vi "例程02-并行转顺序、基于数据流运行.vi"() -> ()   [LabVIEW 2018]
panel:
  out "结果显示 2":dbl
  in  "输入4":dbl
  in  "输入3":dbl
  out "结果显示":dbl
  in  "输入2":dbl
  in  "输入1":dbl
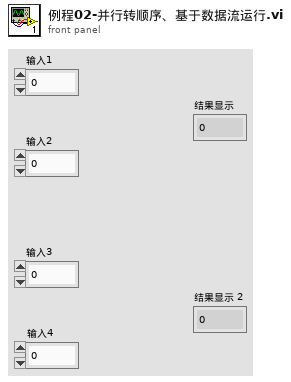
[diagram p1: front panel]
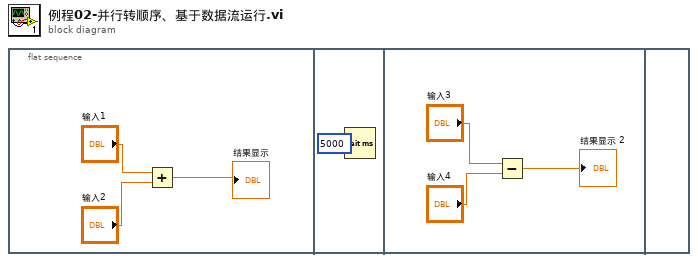
[diagram p0: block diagram]
diagram:
  n1 = flat-sequence {
    frame #0 {
      n2 = Add(x="输入1", y="输入2") -> (x+y=→"结果显示":dbl)
    }
    frame #1 {
      n3 = Wait (ms)(milliseconds to wait=u32 5000 ("等待时间（毫秒）")) -> ()  [unwired: 1 out]
    }
    frame #2 {
      n4 = Subtract(x="输入3", y="输入4") -> (x-y=→"结果显示 2":dbl)
    }
    frame #3 {
    }
  }
